vi "Read Fast.vi"(7 "Type":variant, 8 "error in (no error)":errorcluster, 10 "Name":string, 11 "TwinCAT ADS in":refnum<class "TwinCAT ADS.lvclass">) -> (0 "error out":errorcluster, 1 "Value":variant, 3 "TwinCAT ADS out":refnum<class "TwinCAT ADS.lvclass">)   [LabVIEW 2018, in "TwinCAT ADS.lvclass"]
uses:
  TwinCAT ADS.lvclass
  TwinCAT.Ads
  TwinCAT ADS.lvclass/TwinCAT ADS.ctl
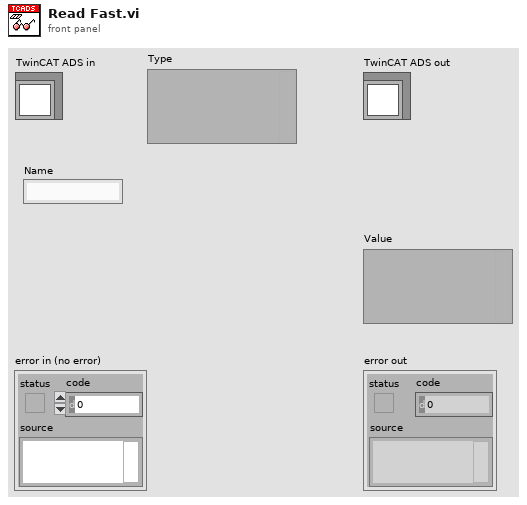
[diagram p1: front panel]
types:
  T1 = typedef "TwinCAT ADS.lvclass/Symbol Information.ctl" = cluster{"Name":string, "Short Name":string, "Size":i32, "Type Category":i32, "Type Name":string, "Type ID":i32, "Index Group":i64, "Index Offset":i64, "Child Count":i32, "Has Rpc Methods?":bool, "Comment":string}
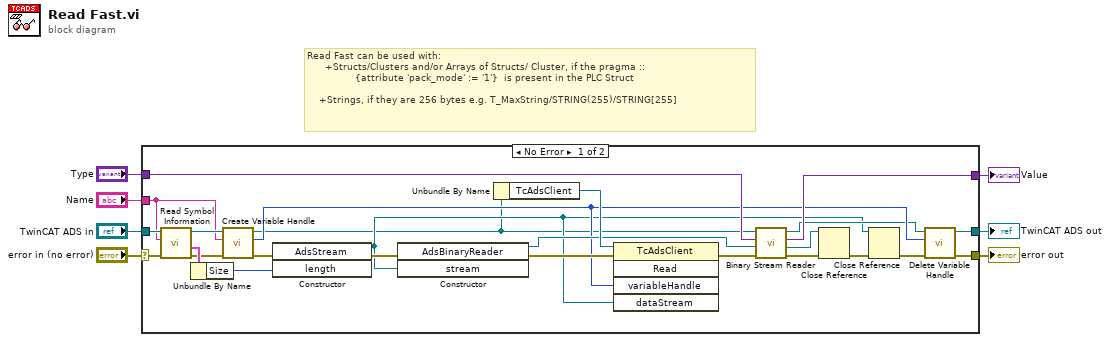
[diagram p0: block diagram]
diagram:
  # "Read Fast can be used with: \n      +Structs/Clusters and/or Arrays of Structs/ Cluster, if the pragma :: \n                {attribute 'pack_mode' := '1'}  is present in the PLC Struct\n\n    +Strings, if they are 256 bytes e.g. T_MaxString/STRING(255)/STRING[255]"
  n1 = case shown="No Error" "error in (no error)" {
    selector: "error in (no error)" -> [w23 w34]
    tunnel: [w14 w34] -> w6
    tunnel: [w15 w33] -> w4
    tunnel: "TwinCAT ADS in" -> [w22 w33]
    tunnel: "Name" -> [w16 _]
    tunnel: [w24 _] -> w2
    tunnel: "Type" -> [w25 _]
    frame No Error {
      n2 = call-dynamic "Read Symbol Information.vi"("error in (no error)"=w23, "Name"=w16, "TwinCAT ADS in"=w22) -> ("error out"=w19:errorcluster, "Symbol Information"=w21:T1, "TwinCAT ADS out"=w18:refnum<class "TwinCAT ADS.lvclass">)  [unwired: 6 in]
      n3 = Unbundle By Name(w21) -> ("Size"=w20:i32)
      n4 = call-dynamic "Create Variable Handle.vi"("error in (no error)"=w19, "Name"=w16, "TwinCAT ADS in"=w18) -> ("error out"=w17:errorcluster, "Handle"=w13:i32, "TwinCAT ADS out"=w8:refnum<class "TwinCAT ADS.lvclass">)  [unwired: 6 in]
      n5 = constructor class="AdsStream"(error in=w17, "length"=w20) -> (reference out=w10:refnum<k24>, error out=w32:errorcluster)  [unwired: 2 in, 2 out]
      n6 = constructor class="AdsBinaryReader"(error in=w32, "stream"=w10) -> (reference out=w28:refnum<k24>, error out=w31:errorcluster)  [unwired: 2 in, 2 out]
      n7 = Unbundle By Name(w8) -> ("TcAdsClient"=w30:refnum<k24>)
      n8 = invoke class="TcAdsClient" method="Read"(reference=w30, error in=w31, "variableHandle"=w13, "dataStream"=w10) -> (error out=w29:errorcluster)  [unwired: 1 in, 4 out]
      n9 = call "Binary Stream Reader.vi"("error in (no error)"=w29, ".NET AdsBinaryReader refnum"=w28, "Type"=w25, "TwinCAT ADS in"=w8) -> ("error out"=w27:errorcluster, ".NET AdsBinaryReader refnum"=w26:refnum<k24>, "Value"=w24:variant, "TwinCAT ADS out"=w11:refnum<class "TwinCAT ADS.lvclass">)  [unwired: 4 in]
      n10 = Close Reference(reference=w26, error in (no error)=w27) -> (error out=w12:errorcluster)
      n11 = Close Reference(reference=w10, error in (no error)=w12) -> (error out=w9:errorcluster)
      n12 = call-dynamic "Delete Variable Handle.vi"("error in (no error)"=w9, "Handle"=w13, "TwinCAT ADS in"=w11) -> ("error out"=w14:errorcluster, "TwinCAT ADS out"=w15:refnum<class "TwinCAT ADS.lvclass">)  [unwired: 7 in]
    }
    frame Error {
    }
  }
  "error out" <- w6
  "TwinCAT ADS out" <- w4
  "Value" <- w2
